vi "Read Variant.vi"(8 "error in (no error)":errorcluster, 11 "SMO.Dictionary.Variant in":refnum<class "SMO.Dictionary.Variant.lvclass">) -> (0 "error out":errorcluster, 2 "Variant":variant, 3 "SMO.Dictionary.Variant out":refnum<class "SMO.Dictionary.Variant.lvclass">)   [LabVIEW 2013, in "SMO.Dictionary.lvlib" / "SMO.Dictionary.Variant.lvclass"]
uses:
  SMO.Dictionary.Variant.lvclass
  SMO.Dictionary.Variant.lvclass/SMO.Dictionary.Variant.ctl
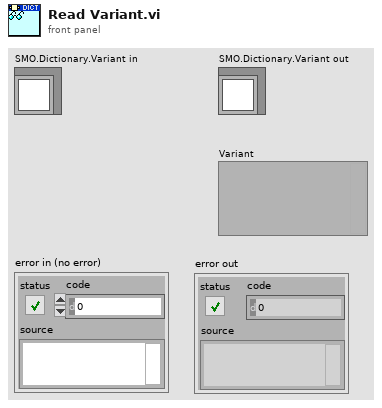
[diagram p1: front panel]
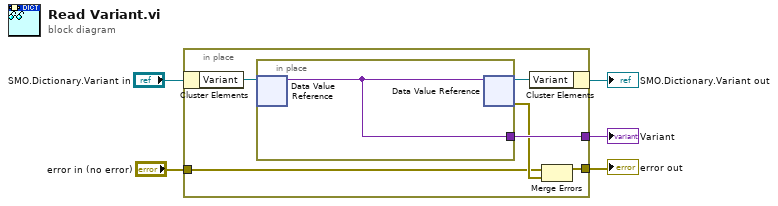
[diagram p0: block diagram]
diagram:
  n1 = in-place {
    in-place-border: [w10] -> w1
    in-place-border: "error in (no error)" -> [w7]
    in-place-border: [w6] -> w2
    n2 = in-place-cluster #1("SMO.Dictionary.Variant in") -> ("Variant"=w11:refnum<data-value>)
    n3 = in-place {
      in-place-border: [w12] -> w10
      n4 = in-place-dvr #2(w11) -> (w12:variant)  [unwired: 1 out]
      n5 = in-place-dvr #2(w12) -> (w9:refnum<data-value>, w8:errorcluster)
    }
    n6 = in-place-cluster #1("Variant"=w9) -> (→"SMO.Dictionary.Variant out":refnum<class "SMO.Dictionary.Variant.lvclass">)
    n7 = Merge Errors(w7, w8) -> (w6:errorcluster)
  }
  "Variant" <- w1
  "error out" <- w2
